vi "S4GUI.vi"(7 "Tab ObsEng":enum32{"Obs", "CCD modes", "Guider", "Eng"}(tab)) -> ()   [LabVIEW 2018] (continued)
        n3988 = call-dynamic "Write AcquisitionC.vi"("error in (no error)"=w9169, "Acquisition.lvclass"=w9171, "S4ACS_GUI in"=w9170) -> ("error out"=w9155:errorcluster, "S4ACS_GUI out"=w9154:refnum<class "S4GUI.lvclass">)  [unwired: 7 in]
      }
      event "Exptime ch4": Value Change {
        n3989 = event-data() -> ("NewVal"=w9178:dbl)  [unwired: 1 in]
        n3990 = call-dynamic "Read AcquisitionD.vi"("error in (no error)"=w9177, "S4ACS_GUI in"=w9176) -> ("error out"=w9192:errorcluster, "Acquisition.lvclass"=w9193:refnum<class "Acquisition.lvclass">, "S4ACS_GUI out"=w9190:refnum<class "S4GUI.lvclass">)  [unwired: 7 in]
        n3991 = call-dynamic "Read Channel.vi"("error in (no error)"=w9192, "Acquisition in"=w9193) -> ("error out"=w9181:errorcluster, "Channel.lvclass"=w9182:refnum<class "Channel.lvclass">, "Acquisition out"=w9183:refnum<class "Acquisition.lvclass">)  [unwired: 7 in]
        n3992 = call-dynamic "Read Interface.vi"("error in (no error)"=w9181, "Channel in"=w9182) -> ("error out"=w9187:errorcluster, "Interface.lvclass"=w9188:refnum<class "Interface.lvclass">, "Channel out"=w9186:refnum<class "Channel.lvclass">)  [unwired: 7 in]
        n3993 = call "Write Exposure Time.vi"("error in (no error)"=w9187, "Exposure Time"=w9178, "Interface in"=w9188) -> ("error out"=w9179:errorcluster, "Interface out"=w9180:refnum<class "Interface.lvclass">)  [unwired: 7 in]
        n3994 = call-dynamic "Write Interface.vi"("error in (no error)"=w9179, "Interface.lvclass"=w9180, "Channel in"=w9186) -> ("error out"=w9185:errorcluster, "Channel out"=w9184:refnum<class "Channel.lvclass">)  [unwired: 7 in]
        n3995 = call-dynamic "Write Channel.vi"("error in (no error)"=w9185, "Channel.lvclass"=w9184, "Acquisition in"=w9183) -> ("error out"=w9189:errorcluster, "Acquisition out"=w9191:refnum<class "Acquisition.lvclass">)  [unwired: 7 in]
        n3996 = call-dynamic "Write AcquisitionD.vi"("error in (no error)"=w9189, "Acquisition.lvclass"=w9191, "S4ACS_GUI in"=w9190) -> ("error out"=w9175:errorcluster, "S4ACS_GUI out"=w9174:refnum<class "S4GUI.lvclass">)  [unwired: 7 in]
      }
      event "Stop ch1": Value Change {
        n3997 = event-data() -> ()  [unwired: 1 in, 6 out]
        n3998 = disable-structure shown="Enabled" {
          disable-tunnel: w9197 -> [w9230 w9258]
          disable-tunnel: w9196 -> [w9228 w9252]
          disable-tunnel: [w9210 w9251] -> w9195
          disable-tunnel: [w9198 w9258] -> w9194
          frame Disabled {
            # "Para movimento \nda lamina retardadora"
            # "Restaura a última sequência de lâminas"
            n3999 = call-dynamic "Read AcquisitionA.vi"("error in (no error)"=w9228, "S4ACS_GUI in"=w9230) -> ("error out"=w9232:errorcluster, "Acquisition.lvclass"=w9231:refnum<class "Acquisition.lvclass">, "S4ACS_GUI out"=w9229:refnum<class "S4GUI.lvclass">)  [unwired: 7 in]
            n4000 = disable-structure shown="Enabled" {
              disable-tunnel: w9232 -> [w9237 w9248]
              disable-tunnel: w9231 -> [w9236 w9249]
              disable-tunnel: [w9234 w9249] -> w9226
              disable-tunnel: [w9233 w9248] -> w9225
              frame Disabled {
                # "Só precisa enviar comando STOP quando\no controle dos ciclos for feito pelo ACS."
                n4001 = call-dynamic "Read Channel.vi"("error in (no error)"=w9237, "Acquisition in"=w9236) -> ("error out"=w9239:errorcluster, "Channel.lvclass"=w9238:refnum<class "Channel.lvclass">, "Acquisition out"=w9245:refnum<class "Acquisition.lvclass">)  [unwired: 7 in]
                n4002 = call-dynamic "Read State Machine.vi"("error in (no error)"=w9239, "Device in"=w9238) -> ("error out"=w9241:errorcluster, "State Machine.lvclass"=w9240:refnum<class "State Machine.lvclass">, "Device out"=w9243:refnum<class "Channel.lvclass">)  [unwired: 7 in]
                n4003 = call "Next State.vi"("error in (no error)"=w9241, "New_State"=u32 70, "State Machine in"=w9240) -> ("error out"=w9244:errorcluster, "State Machine out"=w9242:refnum<class "State Machine.lvclass">)  [unwired: 7 in]
                n4004 = call-dynamic "Write State Machine.vi"("error in (no error)"=w9244, "State Machine.lvclass"=w9242, "Device in"=w9243) -> ("error out"=w9246:errorcluster, "Device out"=w9247:refnum<class "Channel.lvclass">)  [unwired: 7 in]
                n4005 = call-dynamic "Write Channel.vi"("error in (no error)"=w9246, "Channel.lvclass"=w9247, "Acquisition in"=w9245) -> ("error out"=w9233:errorcluster, "Acquisition out"=w9234:refnum<class "Acquisition.lvclass">)  [unwired: 7 in]
              }
              frame Enabled {
                # "Não precisa enviar comando STOP para o ACS\nenquanto o controle dos ciclos for feito pela GUI."
              }
            }
            n4006 = call-dynamic "Write Acq_state.vi"("error in (no error)"=w9225, "Acq_state"=u32 0, "Acquisition in"=w9226) -> ("error out"=w9224:errorcluster, "Acquisition out"=w9223:refnum<class "Acquisition.lvclass">)  [unwired: 7 in]
            n4007 = call-dynamic "Write AcquisitionA.vi"("error in (no error)"=w9224, "Acquisition.lvclass"=w9223, "S4ACS_GUI in"=w9229) -> ("error out"=w9211:errorcluster, "S4ACS_GUI out"=w9209:refnum<class "S4GUI.lvclass">)  [unwired: 7 in]
            n4008 = call "Read Instrument.lvclass.vi"("error in (no error)"=w9211, "S4ACS_GUI in"=w9209) -> ("error out"=w9218:errorcluster, "Instrument.lvclass"=w9221:refnum<class "Instrument.lvclass">, "S4ACS_GUI out"=w9222:refnum<class "S4GUI.lvclass">)  [unwired: 7 in]
            n4009 = call "Read WPROT.vi"("error in (no error)"=w9218, "Instrument in"=w9221) -> ("error out"=w9217:errorcluster, "Opt_Selector.lvclass"=w9219:refnum<class "Opt_Selector.lvclass">, "Instrument out"=w9220:refnum<class "Instrument.lvclass">)  [unwired: 7 in]
            n4010 = call-dynamic "Read sequencia_ant.vi"("error in (no error)"=w9217, "Opt_Selector in"=w9219) -> ("error out"=w9213:errorcluster, "sequencia_ant"=w9212:u16, "Opt_Selector out"=w9214:refnum<class "Opt_Selector.lvclass">)  [unwired: 7 in]
            n4011 = call-dynamic "Write sequencia.vi"("error in (no error)"=w9213, "sequencia"=w9212, "Opt_Selector in"=w9214) -> ("error out"=w9200:errorcluster, "Opt_Selector out"=w9203:refnum<class "Opt_Selector.lvclass">)  [unwired: 7 in]
            n4012 = call-dynamic "Read State Machine.vi"("error in (no error)"=w9200, "Device in"=w9203) -> ("error out"=w9205:errorcluster, "State Machine.lvclass"=w9208:refnum<class "State Machine.lvclass">, "Device out"=w9202:refnum<class "Opt_Selector.lvclass">)  [unwired: 7 in]
            n4013 = call "Next State.vi"("error in (no error)"=w9205, "New_State"=10, "State Machine in"=w9208) -> ("error out"=w9204:errorcluster, "State Machine out"=w9207:refnum<class "State Machine.lvclass">)  [unwired: 7 in]
            n4014 = call-dynamic "Write State Machine.vi"("error in (no error)"=w9204, "State Machine.lvclass"=w9207, "Device in"=w9202) -> ("error out"=w9199:errorcluster, "Device out"=w9201:refnum<class "Opt_Selector.lvclass">)  [unwired: 7 in]
            n4015 = call "Write WPROT.vi"("error in (no error)"=w9199, "Opt_Selector.lvclass"=w9201, "Instrument in"=w9220) -> ("error out"=w9216:errorcluster, "Instrument out"=w9215:refnum<class "Instrument.lvclass">)  [unwired: 7 in]
            n4016 = call "Write Instrument.lvclass.vi"("error in (no error)"=w9216, "Instrument.lvclass"=w9215, "S4ACS_GUI in"=w9222) -> ("error out"=w9210:errorcluster, "S4ACS_GUI out"=w9198:refnum<class "S4GUI.lvclass">)  [unwired: 7 in]
          }
          frame Enabled {
            w9254 = FALSE ("Wait Until Done")
            n4017 = call <vilib>:"Application Directory.vi"() -> ("Application Directory"=w9250:path)
            n4018 = Build Path(base path=w9250, name or relative path="MsgStop1.vi") -> (appended path=w9257:path)
            n4019 = Open VI Reference(vi path=w9257, error in (no error)=w9252) -> (vi reference=w9256:refnum<vi>, error out=w9255:errorcluster)  [unwired: 4 in]
            n4020 = invoke class="VI" method="Run VI"(reference=w9256, error in=w9255, "Wait until done"=w9254, "Auto Dispose Ref"=w9254) -> (error out=w9251:errorcluster)  [unwired: 1 in, 4 out]
          }
        }
      }
      event "Stop ch2": Value Change {
        n4021 = event-data() -> ()  [unwired: 1 in, 6 out]
        n4022 = disable-structure shown="Enabled" {
          disable-tunnel: w9262 -> [w9295 w9316]
          disable-tunnel: w9261 -> [w9293 w9318]
          disable-tunnel: [w9275 w9317] -> w9260
          disable-tunnel: [w9263 w9316] -> w9259
          frame Disabled {
            # "Para movimento \nda lamina retardadora"
            # "Restaura a última sequência de lâminas"
            n4023 = call "Read AcquisitionB.vi"("error in (no error)"=w9293, "S4ACS_GUI in"=w9295) -> ("error out"=w9297:errorcluster, "Acquisition.lvclass"=w9296:refnum<class "Acquisition.lvclass">, "S4ACS_GUI out"=w9294:refnum<class "S4GUI.lvclass">)  [unwired: 7 in]
            n4024 = disable-structure shown="Enabled" {
              disable-tunnel: w9297 -> [w9302 w9313]
              disable-tunnel: w9296 -> [w9301 w9314]
              disable-tunnel: [w9299 w9314] -> w9291
              disable-tunnel: [w9298 w9313] -> w9290
              frame Disabled {
                # "Só precisa enviar comando STOP quando\no controle dos ciclos for feito pelo ACS."
                n4025 = call-dynamic "Read Channel.vi"("error in (no error)"=w9302, "Acquisition in"=w9301) -> ("error out"=w9304:errorcluster, "Channel.lvclass"=w9303:refnum<class "Channel.lvclass">, "Acquisition out"=w9310:refnum<class "Acquisition.lvclass">)  [unwired: 7 in]
                n4026 = call-dynamic "Read State Machine.vi"("error in (no error)"=w9304, "Device in"=w9303) -> ("error out"=w9306:errorcluster, "State Machine.lvclass"=w9305:refnum<class "State Machine.lvclass">, "Device out"=w9308:refnum<class "Channel.lvclass">)  [unwired: 7 in]
                n4027 = call "Next State.vi"("error in (no error)"=w9306, "New_State"=u32 70, "State Machine in"=w9305) -> ("error out"=w9309:errorcluster, "State Machine out"=w9307:refnum<class "State Machine.lvclass">)  [unwired: 7 in]
                n4028 = call-dynamic "Write State Machine.vi"("error in (no error)"=w9309, "State Machine.lvclass"=w9307, "Device in"=w9308) -> ("error out"=w9311:errorcluster, "Device out"=w9312:refnum<class "Channel.lvclass">)  [unwired: 7 in]
                n4029 = call-dynamic "Write Channel.vi"("error in (no error)"=w9311, "Channel.lvclass"=w9312, "Acquisition in"=w9310) -> ("error out"=w9298:errorcluster, "Acquisition out"=w9299:refnum<class "Acquisition.lvclass">)  [unwired: 7 in]
              }
              frame Enabled {
                # "Não precisa enviar comando STOP para o ACS\nenquanto o controle dos ciclos for feito pela GUI."
              }
            }
            n4030 = call-dynamic "Write Acq_state.vi"("error in (no error)"=w9290, "Acq_state"=u32 0, "Acquisition in"=w9291) -> ("error out"=w9289:errorcluster, "Acquisition out"=w9288:refnum<class "Acquisition.lvclass">)  [unwired: 7 in]
            n4031 = call "Write AcquisitionB.vi"("error in (no error)"=w9289, "Acquisition.lvclass"=w9288, "S4ACS_GUI in"=w9294) -> ("error out"=w9276:errorcluster, "S4ACS_GUI out"=w9274:refnum<class "S4GUI.lvclass">)  [unwired: 7 in]
            n4032 = call "Read Instrument.lvclass.vi"("error in (no error)"=w9276, "S4ACS_GUI in"=w9274) -> ("error out"=w9283:errorcluster, "Instrument.lvclass"=w9286:refnum<class "Instrument.lvclass">, "S4ACS_GUI out"=w9287:refnum<class "S4GUI.lvclass">)  [unwired: 7 in]
            n4033 = call "Read WPROT.vi"("error in (no error)"=w9283, "Instrument in"=w9286) -> ("error out"=w9282:errorcluster, "Opt_Selector.lvclass"=w9284:refnum<class "Opt_Selector.lvclass">, "Instrument out"=w9285:refnum<class "Instrument.lvclass">)  [unwired: 7 in]
            n4034 = call-dynamic "Read sequencia_ant.vi"("error in (no error)"=w9282, "Opt_Selector in"=w9284) -> ("error out"=w9278:errorcluster, "sequencia_ant"=w9277:u16, "Opt_Selector out"=w9279:refnum<class "Opt_Selector.lvclass">)  [unwired: 7 in]
            n4035 = call-dynamic "Write sequencia.vi"("error in (no error)"=w9278, "sequencia"=w9277, "Opt_Selector in"=w9279) -> ("error out"=w9265:errorcluster, "Opt_Selector out"=w9268:refnum<class "Opt_Selector.lvclass">)  [unwired: 7 in]
            n4036 = call-dynamic "Read State Machine.vi"("error in (no error)"=w9265, "Device in"=w9268) -> ("error out"=w9270:errorcluster, "State Machine.lvclass"=w9273:refnum<class "State Machine.lvclass">, "Device out"=w9267:refnum<class "Opt_Selector.lvclass">)  [unwired: 7 in]
            n4037 = call "Next State.vi"("error in (no error)"=w9270, "New_State"=10, "State Machine in"=w9273) -> ("error out"=w9269:errorcluster, "State Machine out"=w9272:refnum<class "State Machine.lvclass">)  [unwired: 7 in]
            n4038 = call-dynamic "Write State Machine.vi"("error in (no error)"=w9269, "State Machine.lvclass"=w9272, "Device in"=w9267) -> ("error out"=w9264:errorcluster, "Device out"=w9266:refnum<class "Opt_Selector.lvclass">)  [unwired: 7 in]
            n4039 = call "Write WPROT.vi"("error in (no error)"=w9264, "Opt_Selector.lvclass"=w9266, "Instrument in"=w9285) -> ("error out"=w9281:errorcluster, "Instrument out"=w9280:refnum<class "Instrument.lvclass">)  [unwired: 7 in]
            n4040 = call "Write Instrument.lvclass.vi"("error in (no error)"=w9281, "Instrument.lvclass"=w9280, "S4ACS_GUI in"=w9287) -> ("error out"=w9275:errorcluster, "S4ACS_GUI out"=w9263:refnum<class "S4GUI.lvclass">)  [unwired: 7 in]
          }
          frame Enabled {
            w9320 = FALSE ("Wait Until Done")
            n4041 = call <vilib>:"Application Directory.vi"() -> ("Application Directory"=w9315:path)
            n4042 = Build Path(base path=w9315, name or relative path="MsgStop2.vi") -> (appended path=w9323:path)
            n4043 = Open VI Reference(vi path=w9323, error in (no error)=w9318) -> (vi reference=w9322:refnum<vi>, error out=w9321:errorcluster)  [unwired: 4 in]
            n4044 = invoke class="VI" method="Run VI"(reference=w9322, error in=w9321, "Wait until done"=w9320, "Auto Dispose Ref"=w9320) -> (error out=w9317:errorcluster)  [unwired: 1 in, 4 out]
          }
        }
      }
      event "Stop ch3": Value Change {
        n4045 = event-data() -> ()  [unwired: 1 in, 6 out]
        n4046 = disable-structure shown="Enabled" {
          disable-tunnel: w9327 -> [w9360 w9381]
          disable-tunnel: w9326 -> [w9358 w9383]
          disable-tunnel: [w9340 w9382] -> w9325
          disable-tunnel: [w9328 w9381] -> w9324
          frame Disabled {
            # "Para movimento \nda lamina retardadora"
            # "Restaura a última sequência de lâminas"
            n4047 = call-dynamic "Read AcquisitionC.vi"("error in (no error)"=w9358, "S4ACS_GUI in"=w9360) -> ("error out"=w9362:errorcluster, "Acquisition.lvclass"=w9361:refnum<class "Acquisition.lvclass">, "S4ACS_GUI out"=w9359:refnum<class "S4GUI.lvclass">)  [unwired: 7 in]
            n4048 = disable-structure shown="Enabled" {
              disable-tunnel: w9362 -> [w9367 w9378]
              disable-tunnel: w9361 -> [w9366 w9379]
              disable-tunnel: [w9364 w9379] -> w9356
              disable-tunnel: [w9363 w9378] -> w9355
              frame Disabled {
                # "Só precisa enviar comando STOP quando\no controle dos ciclos for feito pelo ACS."
                n4049 = call-dynamic "Read Channel.vi"("error in (no error)"=w9367, "Acquisition in"=w9366) -> ("error out"=w9369:errorcluster, "Channel.lvclass"=w9368:refnum<class "Channel.lvclass">, "Acquisition out"=w9375:refnum<class "Acquisition.lvclass">)  [unwired: 7 in]
                n4050 = call-dynamic "Read State Machine.vi"("error in (no error)"=w9369, "Device in"=w9368) -> ("error out"=w9371:errorcluster, "State Machine.lvclass"=w9370:refnum<class "State Machine.lvclass">, "Device out"=w9373:refnum<class "Channel.lvclass">)  [unwired: 7 in]
                n4051 = call "Next State.vi"("error in (no error)"=w9371, "New_State"=u32 70, "State Machine in"=w9370) -> ("error out"=w9374:errorcluster, "State Machine out"=w9372:refnum<class "State Machine.lvclass">)  [unwired: 7 in]
                n4052 = call-dynamic "Write State Machine.vi"("error in (no error)"=w9374, "State Machine.lvclass"=w9372, "Device in"=w9373) -> ("error out"=w9376:errorcluster, "Device out"=w9377:refnum<class "Channel.lvclass">)  [unwired: 7 in]
                n4053 = call-dynamic "Write Channel.vi"("error in (no error)"=w9376, "Channel.lvclass"=w9377, "Acquisition in"=w9375) -> ("error out"=w9363:errorcluster, "Acquisition out"=w9364:refnum<class "Acquisition.lvclass">)  [unwired: 7 in]
              }
              frame Enabled {
                # "Não precisa enviar comando STOP para o ACS\nenquanto o controle dos ciclos for feito pela GUI."
              }
            }
            n4054 = call-dynamic "Write Acq_state.vi"("error in (no error)"=w9355, "Acq_state"=u32 0, "Acquisition in"=w9356) -> ("error out"=w9354:errorcluster, "Acquisition out"=w9353:refnum<class "Acquisition.lvclass">)  [unwired: 7 in]
            n4055 = call-dynamic "Write AcquisitionC.vi"("error in (no error)"=w9354, "Acquisition.lvclass"=w9353, "S4ACS_GUI in"=w9359) -> ("error out"=w9341:errorcluster, "S4ACS_GUI out"=w9339:refnum<class "S4GUI.lvclass">)  [unwired: 7 in]
            n4056 = call "Read Instrument.lvclass.vi"("error in (no error)"=w9341, "S4ACS_GUI in"=w9339) -> ("error out"=w9348:errorcluster, "Instrument.lvclass"=w9351:refnum<class "Instrument.lvclass">, "S4ACS_GUI out"=w9352:refnum<class "S4GUI.lvclass">)  [unwired: 7 in]
            n4057 = call "Read WPROT.vi"("error in (no error)"=w9348, "Instrument in"=w9351) -> ("error out"=w9347:errorcluster, "Opt_Selector.lvclass"=w9349:refnum<class "Opt_Selector.lvclass">, "Instrument out"=w9350:refnum<class "Instrument.lvclass">)  [unwired: 7 in]
            n4058 = call-dynamic "Read sequencia_ant.vi"("error in (no error)"=w9347, "Opt_Selector in"=w9349) -> ("error out"=w9343:errorcluster, "sequencia_ant"=w9342:u16, "Opt_Selector out"=w9344:refnum<class "Opt_Selector.lvclass">)  [unwired: 7 in]
            n4059 = call-dynamic "Write sequencia.vi"("error in (no error)"=w9343, "sequencia"=w9342, "Opt_Selector in"=w9344) -> ("error out"=w9330:errorcluster, "Opt_Selector out"=w9333:refnum<class "Opt_Selector.lvclass">)  [unwired: 7 in]
            n4060 = call-dynamic "Read State Machine.vi"("error in (no error)"=w9330, "Device in"=w9333) -> ("error out"=w9335:errorcluster, "State Machine.lvclass"=w9338:refnum<class "State Machine.lvclass">, "Device out"=w9332:refnum<class "Opt_Selector.lvclass">)  [unwired: 7 in]
            n4061 = call "Next State.vi"("error in (no error)"=w9335, "New_State"=10, "State Machine in"=w9338) -> ("error out"=w9334:errorcluster, "State Machine out"=w9337:refnum<class "State Machine.lvclass">)  [unwired: 7 in]
            n4062 = call-dynamic "Write State Machine.vi"("error in (no error)"=w9334, "State Machine.lvclass"=w9337, "Device in"=w9332) -> ("error out"=w9329:errorcluster, "Device out"=w9331:refnum<class "Opt_Selector.lvclass">)  [unwired: 7 in]
            n4063 = call "Write WPROT.vi"("error in (no error)"=w9329, "Opt_Selector.lvclass"=w9331, "Instrument in"=w9350) -> ("error out"=w9346:errorcluster, "Instrument out"=w9345:refnum<class "Instrument.lvclass">)  [unwired: 7 in]
            n4064 = call "Write Instrument.lvclass.vi"("error in (no error)"=w9346, "Instrument.lvclass"=w9345, "S4ACS_GUI in"=w9352) -> ("error out"=w9340:errorcluster, "S4ACS_GUI out"=w9328:refnum<class "S4GUI.lvclass">)  [unwired: 7 in]
          }
          frame Enabled {
            w9385 = FALSE ("Wait Until Done")
            n4065 = call <vilib>:"Application Directory.vi"() -> ("Application Directory"=w9380:path)
            n4066 = Build Path(base path=w9380, name or relative path="MsgStop3.vi") -> (appended path=w9388:path)
            n4067 = Open VI Reference(vi path=w9388, error in (no error)=w9383) -> (vi reference=w9387:refnum<vi>, error out=w9386:errorcluster)  [unwired: 4 in]
            n4068 = invoke class="VI" method="Run VI"(reference=w9387, error in=w9386, "Wait until done"=w9385, "Auto Dispose Ref"=w9385) -> (error out=w9382:errorcluster)  [unwired: 1 in, 4 out]
          }
        }
      }
      event "Stop ch4": Value Change {
        n4069 = event-data() -> ()  [unwired: 1 in, 6 out]
        n4070 = disable-structure shown="Enabled" {
          disable-tunnel: w9392 -> [w9425 w9446]
          disable-tunnel: w9391 -> [w9423 w9448]
          disable-tunnel: [w9405 w9447] -> w9390
          disable-tunnel: [w9393 w9446] -> w9389
          frame Disabled {
            # "Para movimento \nda lamina retardadora"
            # "Restaura a última sequência de lâminas"
            n4071 = call-dynamic "Read AcquisitionD.vi"("error in (no error)"=w9423, "S4ACS_GUI in"=w9425) -> ("error out"=w9427:errorcluster, "Acquisition.lvclass"=w9426:refnum<class "Acquisition.lvclass">, "S4ACS_GUI out"=w9424:refnum<class "S4GUI.lvclass">)  [unwired: 7 in]
            n4072 = disable-structure shown="Enabled" {
              disable-tunnel: w9427 -> [w9432 w9443]
              disable-tunnel: w9426 -> [w9431 w9444]
              disable-tunnel: [w9429 w9444] -> w9421
              disable-tunnel: [w9428 w9443] -> w9420
              frame Disabled {
                # "Só precisa enviar comando STOP quando\no controle dos ciclos for feito pelo ACS."
                n4073 = call-dynamic "Read Channel.vi"("error in (no error)"=w9432, "Acquisition in"=w9431) -> ("error out"=w9434:errorcluster, "Channel.lvclass"=w9433:refnum<class "Channel.lvclass">, "Acquisition out"=w9440:refnum<class "Acquisition.lvclass">)  [unwired: 7 in]
                n4074 = call-dynamic "Read State Machine.vi"("error in (no error)"=w9434, "Device in"=w9433) -> ("error out"=w9436:errorcluster, "State Machine.lvclass"=w9435:refnum<class "State Machine.lvclass">, "Device out"=w9438:refnum<class "Channel.lvclass">)  [unwired: 7 in]
                n4075 = call "Next State.vi"("error in (no error)"=w9436, "New_State"=u32 70, "State Machine in"=w9435) -> ("error out"=w9439:errorcluster, "State Machine out"=w9437:refnum<class "State Machine.lvclass">)  [unwired: 7 in]
                n4076 = call-dynamic "Write State Machine.vi"("error in (no error)"=w9439, "State Machine.lvclass"=w9437, "Device in"=w9438) -> ("error out"=w9441:errorcluster, "Device out"=w9442:refnum<class "Channel.lvclass">)  [unwired: 7 in]
                n4077 = call-dynamic "Write Channel.vi"("error in (no error)"=w9441, "Channel.lvclass"=w9442, "Acquisition in"=w9440) -> ("error out"=w9428:errorcluster, "Acquisition out"=w9429:refnum<class "Acquisition.lvclass">)  [unwired: 7 in]
              }
              frame Enabled {
                # "Não precisa enviar comando STOP para o ACS\nenquanto o controle dos ciclos for feito pela GUI."
              }
            }
            n4078 = call-dynamic "Write Acq_state.vi"("error in (no error)"=w9420, "Acq_state"=u32 0, "Acquisition in"=w9421) -> ("error out"=w9419:errorcluster, "Acquisition out"=w9418:refnum<class "Acquisition.lvclass">)  [unwired: 7 in]
            n4079 = call-dynamic "Write AcquisitionD.vi"("error in (no error)"=w9419, "Acquisition.lvclass"=w9418, "S4ACS_GUI in"=w9424) -> ("error out"=w9406:errorcluster, "S4ACS_GUI out"=w9404:refnum<class "S4GUI.lvclass">)  [unwired: 7 in]
            n4080 = call "Read Instrument.lvclass.vi"("error in (no error)"=w9406, "S4ACS_GUI in"=w9404) -> ("error out"=w9413:errorcluster, "Instrument.lvclass"=w9416:refnum<class "Instrument.lvclass">, "S4ACS_GUI out"=w9417:refnum<class "S4GUI.lvclass">)  [unwired: 7 in]
            n4081 = call "Read WPROT.vi"("error in (no error)"=w9413, "Instrument in"=w9416) -> ("error out"=w9412:errorcluster, "Opt_Selector.lvclass"=w9414:refnum<class "Opt_Selector.lvclass">, "Instrument out"=w9415:refnum<class "Instrument.lvclass">)  [unwired: 7 in]
            n4082 = call-dynamic "Read sequencia_ant.vi"("error in (no error)"=w9412, "Opt_Selector in"=w9414) -> ("error out"=w9408:errorcluster, "sequencia_ant"=w9407:u16, "Opt_Selector out"=w9409:refnum<class "Opt_Selector.lvclass">)  [unwired: 7 in]
            n4083 = call-dynamic "Write sequencia.vi"("error in (no error)"=w9408, "sequencia"=w9407, "Opt_Selector in"=w9409) -> ("error out"=w9395:errorcluster, "Opt_Selector out"=w9398:refnum<class "Opt_Selector.lvclass">)  [unwired: 7 in]
            n4084 = call-dynamic "Read State Machine.vi"("error in (no error)"=w9395, "Device in"=w9398) -> ("error out"=w9400:errorcluster, "State Machine.lvclass"=w9403:refnum<class "State Machine.lvclass">, "Device out"=w9397:refnum<class "Opt_Selector.lvclass">)  [unwired: 7 in]
            n4085 = call "Next State.vi"("error in (no error)"=w9400, "New_State"=10, "State Machine in"=w9403) -> ("error out"=w9399:errorcluster, "State Machine out"=w9402:refnum<class "State Machine.lvclass">)  [unwired: 7 in]
            n4086 = call-dynamic "Write State Machine.vi"("error in (no error)"=w9399, "State Machine.lvclass"=w9402, "Device in"=w9397) -> ("error out"=w9394:errorcluster, "Device out"=w9396:refnum<class "Opt_Selector.lvclass">)  [unwired: 7 in]
            n4087 = call "Write WPROT.vi"("error in (no error)"=w9394, "Opt_Selector.lvclass"=w9396, "Instrument in"=w9415) -> ("error out"=w9411:errorcluster, "Instrument out"=w9410:refnum<class "Instrument.lvclass">)  [unwired: 7 in]
            n4088 = call "Write Instrument.lvclass.vi"("error in (no error)"=w9411, "Instrument.lvclass"=w9410, "S4ACS_GUI in"=w9417) -> ("error out"=w9405:errorcluster, "S4ACS_GUI out"=w9393:refnum<class "S4GUI.lvclass">)  [unwired: 7 in]
          }
          frame Enabled {
            w9450 = FALSE ("Wait Until Done")
            n4089 = call <vilib>:"Application Directory.vi"() -> ("Application Directory"=w9445:path)
            n4090 = Build Path(base path=w9445, name or relative path="MsgStop4.vi") -> (appended path=w9453:path)
            n4091 = Open VI Reference(vi path=w9453, error in (no error)=w9448) -> (vi reference=w9452:refnum<vi>, error out=w9451:errorcluster)  [unwired: 4 in]
            n4092 = invoke class="VI" method="Run VI"(reference=w9452, error in=w9451, "Wait until done"=w9450, "Auto Dispose Ref"=w9450) -> (error out=w9447:errorcluster)  [unwired: 1 in, 4 out]
          }
        }
      }
      event "Pause ch1": Value Change {
        n4093 = event-data() -> ()  [unwired: 1 in, 6 out]
        n4094 = disable-structure shown="Enabled" {
          disable-tunnel: w9457 -> [w9473 w9485]
          disable-tunnel: [w9471 w9483] -> w9456
          disable-tunnel: w9455 -> [w9470 w9484]
          disable-tunnel: [w9458 w9485] -> w9454
          frame Disabled {
            n4095 = call-dynamic "Read AcquisitionA.vi"("error in (no error)"=w9470, "S4ACS_GUI in"=w9473) -> ("error out"=w9465:errorcluster, "Acquisition.lvclass"=w9464:refnum<class "Acquisition.lvclass">, "S4ACS_GUI out"=w9472:refnum<class "S4GUI.lvclass">)  [unwired: 7 in]
            n4096 = call-dynamic "Read Acq_state.vi"("error in (no error)"=w9465, "Acquisition in"=w9464) -> ("error out"=w9467:errorcluster, "Acq_state"=w9468:u32, "Acquisition out"=w9469:refnum<class "Acquisition.lvclass">)  [unwired: 7 in]
            n4097 = call-dynamic "Write Acq_prevstate.vi"("error in (no error)"=w9467, "Acq_prevstate"=w9468, "Acquisition in"=w9469) -> ("error out"=w9462:errorcluster, "Acquisition out"=w9463:refnum<class "Acquisition.lvclass">)  [unwired: 7 in]
            n4098 = call-dynamic "Write Acq_state.vi"("error in (no error)"=w9462, "Acq_state"=u32 400, "Acquisition in"=w9463) -> ("error out"=w9460:errorcluster, "Acquisition out"=w9461:refnum<class "Acquisition.lvclass">)  [unwired: 7 in]
            n4099 = disable-structure shown="Enabled" {
              disable-tunnel: w9460 -> [w9475 w9481]
              disable-tunnel: [w9474 w9481] -> w9459
              frame Disabled {
                n4100 = property on="Start ch1" class="Bool"(error in=w9475, "BoolText.Text"="RESUME" ("Caption.Text")) -> (error out=w9479:errorcluster)  [unwired: 1 in, 1 out]
                n4101 = property on="Pause ch1" class="Bool"(error in=w9479, "DisabledEnum"=T12."Disabled and Grayed Out" ("Disabled")) -> (error out=w9480:errorcluster)  [unwired: 1 in, 1 out]
                n4102 = property on="Start ch1" class="Bool"(error in=w9480, "DisabledEnum"=T12."Enabled" ("Disabled")) -> (error out=w9474:errorcluster)  [unwired: 1 in, 1 out]
              }
              frame Enabled {
              }
            }
            n4103 = call-dynamic "Write AcquisitionA.vi"("error in (no error)"=w9459, "Acquisition.lvclass"=w9461, "S4ACS_GUI in"=w9472) -> ("error out"=w9471:errorcluster, "S4ACS_GUI out"=w9458:refnum<class "S4GUI.lvclass">)  [unwired: 7 in]
          }
          frame Enabled {
            w9487 = FALSE ("Wait Until Done")
            n4104 = call <vilib>:"Application Directory.vi"() -> ("Application Directory"=w9482:path)
            n4105 = Build Path(base path=w9482, name or relative path="MsgPause1.vi") -> (appended path=w9490:path)
            n4106 = Open VI Reference(vi path=w9490, error in (no error)=w9484) -> (vi reference=w9489:refnum<vi>, error out=w9488:errorcluster)  [unwired: 4 in]
            n4107 = invoke class="VI" method="Run VI"(reference=w9489, error in=w9488, "Wait until done"=w9487, "Auto Dispose Ref"=w9487) -> (error out=w9483:errorcluster)  [unwired: 1 in, 4 out]
          }
        }
      }
      event "Pause ch2": Value Change {
        n4108 = event-data() -> ()  [unwired: 1 in, 6 out]
        n4109 = disable-structure shown="Enabled" {
          disable-tunnel: w9494 -> [w9509 w9511]
          disable-tunnel: [w9507 w9512] -> w9493
          disable-tunnel: w9492 -> [w9506 w9513]
          disable-tunnel: [w9496 w9511] -> w9491
          frame Disabled {
            n4110 = call "Read AcquisitionB.vi"("error in (no error)"=w9506, "S4ACS_GUI in"=w9509) -> ("error out"=w9501:errorcluster, "Acquisition.lvclass"=w9500:refnum<class "Acquisition.lvclass">, "S4ACS_GUI out"=w9508:refnum<class "S4GUI.lvclass">)  [unwired: 7 in]
            n4111 = call-dynamic "Read Acq_state.vi"("error in (no error)"=w9501, "Acquisition in"=w9500) -> ("error out"=w9503:errorcluster, "Acq_state"=w9504:u32, "Acquisition out"=w9505:refnum<class "Acquisition.lvclass">)  [unwired: 7 in]
            n4112 = call-dynamic "Write Acq_prevstate.vi"("error in (no error)"=w9503, "Acq_prevstate"=w9504, "Acquisition in"=w9505) -> ("error out"=w9498:errorcluster, "Acquisition out"=w9499:refnum<class "Acquisition.lvclass">)  [unwired: 7 in]
            n4113 = call-dynamic "Write Acq_state.vi"("error in (no error)"=w9498, "Acq_state"=u32 400, "Acquisition in"=w9499) -> ("error out"=w9495:errorcluster, "Acquisition out"=w9497:refnum<class "Acquisition.lvclass">)  [unwired: 7 in]
            n4114 = call "Write AcquisitionB.vi"("error in (no error)"=w9495, "Acquisition.lvclass"=w9497, "S4ACS_GUI in"=w9508) -> ("error out"=w9507:errorcluster, "S4ACS_GUI out"=w9496:refnum<class "S4GUI.lvclass">)  [unwired: 7 in]
          }
          frame Enabled {
            w9515 = FALSE ("Wait Until Done")
            n4115 = call <vilib>:"Application Directory.vi"() -> ("Application Directory"=w9510:path)
            n4116 = Build Path(base path=w9510, name or relative path="MsgPause2.vi") -> (appended path=w9518:path)
            n4117 = Open VI Reference(vi path=w9518, error in (no error)=w9513) -> (vi reference=w9517:refnum<vi>, error out=w9516:errorcluster)  [unwired: 4 in]
            n4118 = invoke class="VI" method="Run VI"(reference=w9517, error in=w9516, "Wait until done"=w9515, "Auto Dispose Ref"=w9515) -> (error out=w9512:errorcluster)  [unwired: 1 in, 4 out]
          }
        }
      }
      event "Pause ch3": Value Change {
        n4119 = event-data() -> ()  [unwired: 1 in, 6 out]
        n4120 = disable-structure shown="Enabled" {
          disable-tunnel: w9522 -> [w9537 w9539]
          disable-tunnel: [w9535 w9540] -> w9521
          disable-tunnel: w9520 -> [w9534 w9541]
          disable-tunnel: [w9524 w9539] -> w9519
          frame Disabled {
            n4121 = call-dynamic "Read AcquisitionC.vi"("error in (no error)"=w9534, "S4ACS_GUI in"=w9537) -> ("error out"=w9529:errorcluster, "Acquisition.lvclass"=w9528:refnum<class "Acquisition.lvclass">, "S4ACS_GUI out"=w9536:refnum<class "S4GUI.lvclass">)  [unwired: 7 in]
            n4122 = call-dynamic "Read Acq_state.vi"("error in (no error)"=w9529, "Acquisition in"=w9528) -> ("error out"=w9531:errorcluster, "Acq_state"=w9532:u32, "Acquisition out"=w9533:refnum<class "Acquisition.lvclass">)  [unwired: 7 in]
            n4123 = call-dynamic "Write Acq_prevstate.vi"("error in (no error)"=w9531, "Acq_prevstate"=w9532, "Acquisition in"=w9533) -> ("error out"=w9526:errorcluster, "Acquisition out"=w9527:refnum<class "Acquisition.lvclass">)  [unwired: 7 in]
            n4124 = call-dynamic "Write Acq_state.vi"("error in (no error)"=w9526, "Acq_state"=u32 400, "Acquisition in"=w9527) -> ("error out"=w9523:errorcluster, "Acquisition out"=w9525:refnum<class "Acquisition.lvclass">)  [unwired: 7 in]
            n4125 = call-dynamic "Write AcquisitionC.vi"("error in (no error)"=w9523, "Acquisition.lvclass"=w9525, "S4ACS_GUI in"=w9536) -> ("error out"=w9535:errorcluster, "S4ACS_GUI out"=w9524:refnum<class "S4GUI.lvclass">)  [unwired: 7 in]
          }
          frame Enabled {
            w9543 = FALSE ("Wait Until Done")
            n4126 = call <vilib>:"Application Directory.vi"() -> ("Application Directory"=w9538:path)
            n4127 = Build Path(base path=w9538, name or relative path="MsgPause3.vi") -> (appended path=w9546:path)
            n4128 = Open VI Reference(vi path=w9546, error in (no error)=w9541) -> (vi reference=w9545:refnum<vi>, error out=w9544:errorcluster)  [unwired: 4 in]
            n4129 = invoke class="VI" method="Run VI"(reference=w9545, error in=w9544, "Wait until done"=w9543, "Auto Dispose Ref"=w9543) -> (error out=w9540:errorcluster)  [unwired: 1 in, 4 out]
          }
        }
      }
      event "Pause ch4": Value Change {
        n4130 = event-data() -> ()  [unwired: 1 in, 6 out]
        n4131 = disable-structure shown="Enabled" {
          disable-tunnel: w9550 -> [w9565 w9574]
          disable-tunnel: [w9563 w9567] -> w9549
          disable-tunnel: w9548 -> [w9562 w9568]
          disable-tunnel: [w9552 w9574] -> w9547
          frame Disabled {
            n4132 = call-dynamic "Read AcquisitionD.vi"("error in (no error)"=w9562, "S4ACS_GUI in"=w9565) -> ("error out"=w9557:errorcluster, "Acquisition.lvclass"=w9556:refnum<class "Acquisition.lvclass">, "S4ACS_GUI out"=w9564:refnum<class "S4GUI.lvclass">)  [unwired: 7 in]
            n4133 = call-dynamic "Read Acq_state.vi"("error in (no error)"=w9557, "Acquisition in"=w9556) -> ("error out"=w9559:errorcluster, "Acq_state"=w9560:u32, "Acquisition out"=w9561:refnum<class "Acquisition.lvclass">)  [unwired: 7 in]
            n4134 = call-dynamic "Write Acq_prevstate.vi"("error in (no error)"=w9559, "Acq_prevstate"=w9560, "Acquisition in"=w9561) -> ("error out"=w9554:errorcluster, "Acquisition out"=w9555:refnum<class "Acquisition.lvclass">)  [unwired: 7 in]
            n4135 = call-dynamic "Write Acq_state.vi"("error in (no error)"=w9554, "Acq_state"=u32 400, "Acquisition in"=w9555) -> ("error out"=w9551:errorcluster, "Acquisition out"=w9553:refnum<class "Acquisition.lvclass">)  [unwired: 7 in]
            n4136 = call-dynamic "Write AcquisitionD.vi"("error in (no error)"=w9551, "Acquisition.lvclass"=w9553, "S4ACS_GUI in"=w9564) -> ("error out"=w9563:errorcluster, "S4ACS_GUI out"=w9552:refnum<class "S4GUI.lvclass">)  [unwired: 7 in]
          }
          frame Enabled {
            w9570 = FALSE ("Wait Until Done")
            n4137 = call <vilib>:"Application Directory.vi"() -> ("Application Directory"=w9566:path)
            n4138 = Build Path(base path=w9566, name or relative path="MsgPause4.vi") -> (appended path=w9573:path)
            n4139 = Open VI Reference(vi path=w9573, error in (no error)=w9568) -> (vi reference=w9572:refnum<vi>, error out=w9571:errorcluster)  [unwired: 4 in]
            n4140 = invoke class="VI" method="Run VI"(reference=w9572, error in=w9571, "Wait until done"=w9570, "Auto Dispose Ref"=w9570) -> (error out=w9567:errorcluster)  [unwired: 1 in, 4 out]
          }
        }
      }
      event "Stop SM": Value Change {
        w9580 = 0.0 ("Scale.Range:Minor Increment")
        n4141 = event-data() -> ()  [unwired: 1 in, 6 out]
        n4142 = call-dynamic "Write User Event.vi"("error in (no error)"=w9578, "User Event"="STOP SM CLICKED", "S4GUI in"=w9579) -> ("error out"=w9576:errorcluster, "S4GUI out"=w9577:refnum<class "S4GUI.lvclass">)  [unwired: 7 in]
        n4143 = disable-structure shown="Enabled" {
          disable-tunnel: w9577 -> [w9617 w9641]
          disable-tunnel: w9576 -> [w9615 w9642]
          disable-tunnel: [w9602 w9640] -> w9582
          disable-tunnel: [w9586 w9641] -> w9581
          frame Disabled {
            # "Não precisa enviar comando STOP para o ACS\nenquanto o controle dos ciclos for feito pela GUI."
            # "Para movimento \nda lamina retardadora"
            # "Restaura a sequencia anterior"
            n4144 = call-dynamic "Read AcquisitionA.vi"("error in (no error)"=w9615, "S4ACS_GUI in"=w9617) -> ("error out"=w9619:errorcluster, "Acquisition.lvclass"=w9618:refnum<class "Acquisition.lvclass">, "S4ACS_GUI out"=w9616:refnum<class "S4GUI.lvclass">)  [unwired: 7 in]
            n4145 = disable-structure shown="Enabled" {
              disable-tunnel: [w9633 w9637] -> w9621
              disable-tunnel: [w9632 w9638] -> w9620
              disable-tunnel: w9619 -> [w9624 w9637]
              disable-tunnel: w9618 -> [w9623 w9638]
              frame Disabled {
                n4146 = call-dynamic "Read Channel.vi"("error in (no error)"=w9624, "Acquisition in"=w9623) -> ("error out"=w9626:errorcluster, "Channel.lvclass"=w9625:refnum<class "Channel.lvclass">, "Acquisition out"=w9634:refnum<class "Acquisition.lvclass">)  [unwired: 7 in]
                n4147 = call-dynamic "Read State Machine.vi"("error in (no error)"=w9626, "Device in"=w9625) -> ("error out"=w9628:errorcluster, "State Machine.lvclass"=w9627:refnum<class "State Machine.lvclass">, "Device out"=w9630:refnum<class "Channel.lvclass">)  [unwired: 7 in]
                n4148 = call "Next State.vi"("error in (no error)"=w9628, "New_State"=u32 70, "State Machine in"=w9627) -> ("error out"=w9631:errorcluster, "State Machine out"=w9629:refnum<class "State Machine.lvclass">)  [unwired: 7 in]
                n4149 = call-dynamic "Write State Machine.vi"("error in (no error)"=w9631, "State Machine.lvclass"=w9629, "Device in"=w9630) -> ("error out"=w9635:errorcluster, "Device out"=w9636:refnum<class "Channel.lvclass">)  [unwired: 7 in]
                n4150 = call-dynamic "Write Channel.vi"("error in (no error)"=w9635, "Channel.lvclass"=w9636, "Acquisition in"=w9634) -> ("error out"=w9633:errorcluster, "Acquisition out"=w9632:refnum<class "Acquisition.lvclass">)  [unwired: 7 in]
              }
              frame Enabled {
              }
            }
            n4151 = call-dynamic "Write AcquisitionA.vi"("error in (no error)"=w9621, "Acquisition.lvclass"=w9620, "S4ACS_GUI in"=w9616) -> ("error out"=w9584:errorcluster, "S4ACS_GUI out"=w9585:refnum<class "S4GUI.lvclass">)  [unwired: 7 in]
            n4152 = call-dynamic "Write Obs_state.vi"("error in (no error)"=w9584, "Obs_state"=u32 0, "S4ACS_GUI in"=w9585) -> ("error out"=w9604:errorcluster, "S4ACS_GUI out"=w9605:refnum<class "S4GUI.lvclass">)  [unwired: 7 in]
            n4153 = call "Read Instrument.lvclass.vi"("error in (no error)"=w9604, "S4ACS_GUI in"=w9605) -> ("error out"=w9613:errorcluster, "Instrument.lvclass"=w9611:refnum<class "Instrument.lvclass">, "S4ACS_GUI out"=w9612:refnum<class "S4GUI.lvclass">)  [unwired: 7 in]
            n4154 = call "Read WPROT.vi"("error in (no error)"=w9613, "Instrument in"=w9611) -> ("error out"=w9598:errorcluster, "Opt_Selector.lvclass"=w9601:refnum<class "Opt_Selector.lvclass">, "Instrument out"=w9610:refnum<class "Instrument.lvclass">)  [unwired: 7 in]
            n4155 = call-dynamic "Read sequencia_ant.vi"("error in (no error)"=w9598, "Opt_Selector in"=w9601) -> ("error out"=w9597:errorcluster, "sequencia_ant"=w9599:u16, "Opt_Selector out"=w9600:refnum<class "Opt_Selector.lvclass">)  [unwired: 7 in]
            n4156 = call-dynamic "Write sequencia.vi"("error in (no error)"=w9597, "sequencia"=w9599, "Opt_Selector in"=w9600) -> ("error out"=w9595:errorcluster, "Opt_Selector out"=w9596:refnum<class "Opt_Selector.lvclass">)  [unwired: 7 in]
            n4157 = call-dynamic "Read State Machine.vi"("error in (no error)"=w9595, "Device in"=w9596) -> ("error out"=w9590:errorcluster, "State Machine.lvclass"=w9593:refnum<class "State Machine.lvclass">, "Device out"=w9594:refnum<class "Opt_Selector.lvclass">)  [unwired: 7 in]
            n4158 = call "Next State.vi"("error in (no error)"=w9590, "New_State"=10, "State Machine in"=w9593) -> ("error out"=w9589:errorcluster, "State Machine out"=w9592:refnum<class "State Machine.lvclass">)  [unwired: 7 in]
            n4159 = call-dynamic "Write State Machine.vi"("error in (no error)"=w9589, "State Machine.lvclass"=w9592, "Device in"=w9594) -> ("error out"=w9588:errorcluster, "Device out"=w9587:refnum<class "Opt_Selector.lvclass">)  [unwired: 7 in]
            n4160 = call "Write WPROT.vi"("error in (no error)"=w9588, "Opt_Selector.lvclass"=w9587, "Instrument in"=w9610) -> ("error out"=w9608:errorcluster, "Instrument out"=w9609:refnum<class "Instrument.lvclass">)  [unwired: 7 in]
            n4161 = call "Write Instrument.lvclass.vi"("error in (no error)"=w9608, "Instrument.lvclass"=w9609, "S4ACS_GUI in"=w9612) -> ("error out"=w9607:errorcluster, "S4ACS_GUI out"=w9606:refnum<class "S4GUI.lvclass">)  [unwired: 7 in]
            n4162 = call-dynamic "Write ciclos.vi"("error in (no error)"=w9607, "ciclos"=u32 0, "S4ACS_GUI in"=w9606) -> ("error out"=w9602:errorcluster, "S4ACS_GUI out"=w9586:refnum<class "S4GUI.lvclass">)  [unwired: 7 in]
          }
          frame Enabled {
            w9644 = FALSE ("Wait Until Done")
            n4163 = call <vilib>:"Application Directory.vi"() -> ("Application Directory"=w9639:path)
            n4164 = Build Path(base path=w9639, name or relative path="MsgStopSync.vi") -> (appended path=w9647:path)
            n4165 = Open VI Reference(vi path=w9647, error in (no error)=w9642) -> (vi reference=w9646:refnum<vi>, error out=w9645:errorcluster)  [unwired: 4 in]
            n4166 = invoke class="VI" method="Run VI"(reference=w9646, error in=w9645, "Wait until done"=w9644, "Auto Dispose Ref"=w9644) -> (error out=w9640:errorcluster)  [unwired: 1 in, 4 out]
          }
        }
        n4167 = property on="#Cycles Done" class="Slide (strict)"(error in=w9582, "Scale.Maximum"=w9580, "Scale.Minimum"=w9580) -> (error out=w9583:errorcluster)  [unwired: 1 in, 1 out]
      }
      event "Abort SM": Value Change {
        w9655 = 0.0 ("Scale.Range:Minor Increment")
        n4168 = event-data() -> ()  [unwired: 1 in, 6 out]
        n4169 = call-dynamic "Write User Event.vi"("error in (no error)"=w9651, "User Event"="ABORT SM CLICKED", "S4GUI in"=w9652) -> ("error out"=w9649:errorcluster, "S4GUI out"=w9650:refnum<class "S4GUI.lvclass">)  [unwired: 7 in]
        n4170 = disable-structure shown="Enabled" {
          disable-tunnel: w9650 -> [w9746 w9770]
          disable-tunnel: w9649 -> [w9744 w9772]
          disable-tunnel: [w9658 w9770] -> w9654
          disable-tunnel: [w9657 w9771] -> w9653
          frame Disabled {
            # "Restaura a sequencia anterior"
            # "Para movimento \nda lamina retardadora"
            n4171 = call-dynamic "Read AcquisitionA.vi"("error in (no error)"=w9744, "S4ACS_GUI in"=w9746) -> ("error out"=w9749:errorcluster, "Acquisition.lvclass"=w9748:refnum<class "Acquisition.lvclass">, "S4ACS_GUI out"=w9745:refnum<class "S4GUI.lvclass">)  [unwired: 7 in]
            n4172 = call-dynamic "Read Channel.vi"("error in (no error)"=w9749, "Acquisition in"=w9748) -> ("error out"=w9751:errorcluster, "Channel.lvclass"=w9750:refnum<class "Channel.lvclass">, "Acquisition out"=w9759:refnum<class "Acquisition.lvclass">)  [unwired: 7 in]
            n4173 = call-dynamic "Read State Machine.vi"("error in (no error)"=w9751, "Device in"=w9750) -> ("error out"=w9753:errorcluster, "State Machine.lvclass"=w9752:refnum<class "State Machine.lvclass">, "Device out"=w9755:refnum<class "Channel.lvclass">)  [unwired: 7 in]
            n4174 = call "Next State.vi"("error in (no error)"=w9753, "New_State"=u32 80, "State Machine in"=w9752) -> ("error out"=w9756:errorcluster, "State Machine out"=w9754:refnum<class "State Machine.lvclass">)  [unwired: 7 in]
            n4175 = call-dynamic "Write State Machine.vi"("error in (no error)"=w9756, "State Machine.lvclass"=w9754, "Device in"=w9755) -> ("error out"=w9760:errorcluster, "Device out"=w9761:refnum<class "Channel.lvclass">)  [unwired: 7 in]
            n4176 = call-dynamic "Write Channel.vi"("error in (no error)"=w9760, "Channel.lvclass"=w9761, "Acquisition in"=w9759) -> ("error out"=w9758:errorcluster, "Acquisition out"=w9757:refnum<class "Acquisition.lvclass">)  [unwired: 7 in]
            n4177 = call-dynamic "Write AcquisitionA.vi"("error in (no error)"=w9758, "Acquisition.lvclass"=w9757, "S4ACS_GUI in"=w9745) -> ("error out"=w9730:errorcluster, "S4ACS_GUI out"=w9729:refnum<class "S4GUI.lvclass">)  [unwired: 7 in]
            n4178 = call "Read AcquisitionB.vi"("error in (no error)"=w9730, "S4ACS_GUI in"=w9729) -> ("error out"=w9723:errorcluster, "Acquisition.lvclass"=w9727:refnum<class "Acquisition.lvclass">, "S4ACS_GUI out"=w9728:refnum<class "S4GUI.lvclass">)  [unwired: 7 in]
            n4179 = call-dynamic "Read Channel.vi"("error in (no error)"=w9723, "Acquisition in"=w9727) -> ("error out"=w9738:errorcluster, "Channel.lvclass"=w9739:refnum<class "Channel.lvclass">, "Acquisition out"=w9725:refnum<class "Acquisition.lvclass">)  [unwired: 7 in]
            n4180 = call-dynamic "Read State Machine.vi"("error in (no error)"=w9738, "Device in"=w9739) -> ("error out"=w9736:errorcluster, "State Machine.lvclass"=w9737:refnum<class "State Machine.lvclass">, "Device out"=w9734:refnum<class "Channel.lvclass">)  [unwired: 7 in]
            n4181 = call "Next State.vi"("error in (no error)"=w9736, "New_State"=u32 80, "State Machine in"=w9737) -> ("error out"=w9733:errorcluster, "State Machine out"=w9735:refnum<class "State Machine.lvclass">)  [unwired: 7 in]
            n4182 = call-dynamic "Write State Machine.vi"("error in (no error)"=w9733, "State Machine.lvclass"=w9735, "Device in"=w9734) -> ("error out"=w9732:errorcluster, "Device out"=w9731:refnum<class "Channel.lvclass">)  [unwired: 7 in]
            n4183 = call-dynamic "Write Channel.vi"("error in (no error)"=w9732, "Channel.lvclass"=w9731, "Acquisition in"=w9725) -> ("error out"=w9724:errorcluster, "Acquisition out"=w9726:refnum<class "Acquisition.lvclass">)  [unwired: 7 in]
            n4184 = call "Write AcquisitionB.vi"("error in (no error)"=w9724, "Acquisition.lvclass"=w9726, "S4ACS_GUI in"=w9728) -> ("error out"=w9690:errorcluster, "S4ACS_GUI out"=w9689:refnum<class "S4GUI.lvclass">)  [unwired: 7 in]
            n4185 = call-dynamic "Read AcquisitionC.vi"("error in (no error)"=w9690, "S4ACS_GUI in"=w9689) -> ("error out"=w9707:errorcluster, "Acquisition.lvclass"=w9711:refnum<class "Acquisition.lvclass">, "S4ACS_GUI out"=w9712:refnum<class "S4GUI.lvclass">)  [unwired: 7 in]
            n4186 = call-dynamic "Read Channel.vi"("error in (no error)"=w9707, "Acquisition in"=w9711) -> ("error out"=w9720:errorcluster, "Channel.lvclass"=w9721:refnum<class "Channel.lvclass">, "Acquisition out"=w9709:refnum<class "Acquisition.lvclass">)  [unwired: 7 in]
            n4187 = call-dynamic "Read State Machine.vi"("error in (no error)"=w9720, "Device in"=w9721) -> ("error out"=w9718:errorcluster, "State Machine.lvclass"=w9719:refnum<class "State Machine.lvclass">, "Device out"=w9716:refnum<class "Channel.lvclass">)  [unwired: 7 in]
            n4188 = call "Next State.vi"("error in (no error)"=w9718, "New_State"=u32 80, "State Machine in"=w9719) -> ("error out"=w9715:errorcluster, "State Machine out"=w9717:refnum<class "State Machine.lvclass">)  [unwired: 7 in]
            n4189 = call-dynamic "Write State Machine.vi"("error in (no error)"=w9715, "State Machine.lvclass"=w9717, "Device in"=w9716) -> ("error out"=w9714:errorcluster, "Device out"=w9713:refnum<class "Channel.lvclass">)  [unwired: 7 in]
            n4190 = call-dynamic "Write Channel.vi"("error in (no error)"=w9714, "Channel.lvclass"=w9713, "Acquisition in"=w9709) -> ("error out"=w9708:errorcluster, "Acquisition out"=w9710:refnum<class "Acquisition.lvclass">)  [unwired: 7 in]
            n4191 = call-dynamic "Write AcquisitionC.vi"("error in (no error)"=w9708, "Acquisition.lvclass"=w9710, "S4ACS_GUI in"=w9712) -> ("error out"=w9688:errorcluster, "S4ACS_GUI out"=w9687:refnum<class "S4GUI.lvclass">)  [unwired: 7 in]
            n4192 = call-dynamic "Read AcquisitionD.vi"("error in (no error)"=w9688, "S4ACS_GUI in"=w9687) -> ("error out"=w9691:errorcluster, "Acquisition.lvclass"=w9695:refnum<class "Acquisition.lvclass">, "S4ACS_GUI out"=w9696:refnum<class "S4GUI.lvclass">)  [unwired: 7 in]
            n4193 = call-dynamic "Read Channel.vi"("error in (no error)"=w9691, "Acquisition in"=w9695) -> ("error out"=w9704:errorcluster, "Channel.lvclass"=w9705:refnum<class "Channel.lvclass">, "Acquisition out"=w9693:refnum<class "Acquisition.lvclass">)  [unwired: 7 in]
            n4194 = call-dynamic "Read State Machine.vi"("error in (no error)"=w9704, "Device in"=w9705) -> ("error out"=w9702:errorcluster, "State Machine.lvclass"=w9703:refnum<class "State Machine.lvclass">, "Device out"=w9700:refnum<class "Channel.lvclass">)  [unwired: 7 in]
            n4195 = call "Next State.vi"("error in (no error)"=w9702, "New_State"=u32 80, "State Machine in"=w9703) -> ("error out"=w9699:errorcluster, "State Machine out"=w9701:refnum<class "State Machine.lvclass">)  [unwired: 7 in]
            n4196 = call-dynamic "Write State Machine.vi"("error in (no error)"=w9699, "State Machine.lvclass"=w9701, "Device in"=w9700) -> ("error out"=w9698:errorcluster, "Device out"=w9697:refnum<class "Channel.lvclass">)  [unwired: 7 in]
            n4197 = call-dynamic "Write Channel.vi"("error in (no error)"=w9698, "Channel.lvclass"=w9697, "Acquisition in"=w9693) -> ("error out"=w9692:errorcluster, "Acquisition out"=w9694:refnum<class "Acquisition.lvclass">)  [unwired: 7 in]
            n4198 = call-dynamic "Write AcquisitionD.vi"("error in (no error)"=w9692, "Acquisition.lvclass"=w9694, "S4ACS_GUI in"=w9696) -> ("error out"=w9685:errorcluster, "S4ACS_GUI out"=w9686:refnum<class "S4GUI.lvclass">)  [unwired: 7 in]
            n4199 = disable-structure shown="Enabled" {
              disable-tunnel: w9686 -> [w9766 w9768]
              disable-tunnel: w9685 -> [w9765 w9767]
              disable-tunnel: [w9763 w9768] -> w9742
              disable-tunnel: [w9762 w9767] -> w9741
              frame Disabled {
                n4200 = call-dynamic "Write aborted.vi"("error in (no error)"=w9765, "aborted"=TRUE ("stopped"), "S4ACS_GUI in"=w9766) -> ("error out"=w9762:errorcluster, "S4ACS_GUI out"=w9763:refnum<class "S4GUI.lvclass">)  [unwired: 7 in]
              }
              frame Enabled {
              }
            }
            n4201 = call-dynamic "Write Obs_state.vi"("error in (no error)"=w9741, "Obs_state"=u32 0, "S4ACS_GUI in"=w9742) -> ("error out"=w9659:errorcluster, "S4ACS_GUI out"=w9660:refnum<class "S4GUI.lvclass">)  [unwired: 7 in]
            n4202 = call "Read Instrument.lvclass.vi"("error in (no error)"=w9659, "S4ACS_GUI in"=w9660) -> ("error out"=w9679:errorcluster, "Instrument.lvclass"=w9681:refnum<class "Instrument.lvclass">, "S4ACS_GUI out"=w9680:refnum<class "S4GUI.lvclass">)  [unwired: 7 in]
